vi "subvii.vi"() -> ()   [LabVIEW 2011]
panel:
  out "Numeric":dbl
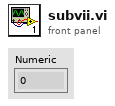
[diagram p1: front panel]
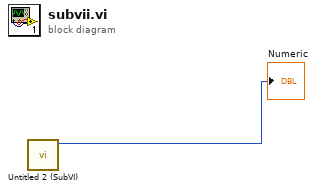
[diagram p0: block diagram]
diagram:
  n1 = call "Untitled 2 (SubVI).vi"() -> ("Numeric"=→"Numeric":i32)  [unwired: 11 in]
